vi "AutoWfmToSpreadsheet.vi"() -> ()   [LabVIEW 2017]
uses:
  <vilib>/Waveform/WDTOps.llb/WDT Scale Delta t DBL.vi
  <vilib>/Waveform/WDTFileIO.llb/Read Waveform from File.vi
  <vilib>/Waveform/WDTOps.llb/WDT Index Channel DBL.vi
  <vilib>/measure/maspectr.llb/FFT Power Spectrum and PSD for 1 Chan.vi
  <vilib>/Waveform/WDTFileIO.llb/Export Waveforms To Spreadsheet File (1D).vi
  <vilib>/measure/NI_MAPro.lvlib
panel:
  out "POWER":dbl[](graph)
  out "?":string
  out "Sinal adquirido":waveform(dbl)(graph)
  in  "?":bool
  in  "Escolher arquivo":i32
  out "Sinal de Referência":waveform(dbl)(graph)
  in  "Exportar":bool
  out "result string":string
  in  "Local da pasta com arquivos wfm":path=path "C:/Users/lucas/Documents/GitHub/INT/Novo Ensaio US/NOVOS_SINAIS/sinais/wfm"
  out "element":string
  out "Visualizar":i32
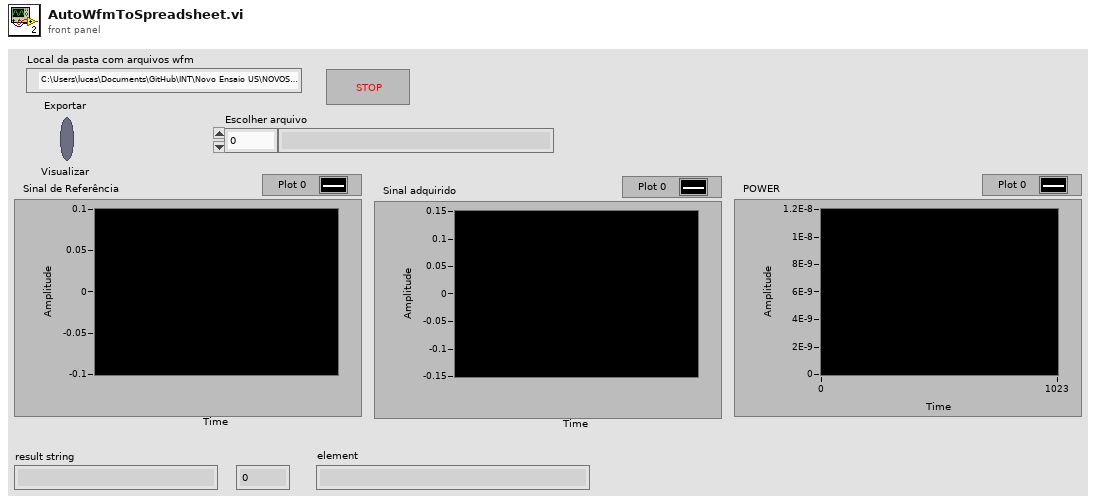
[diagram p1: front panel]
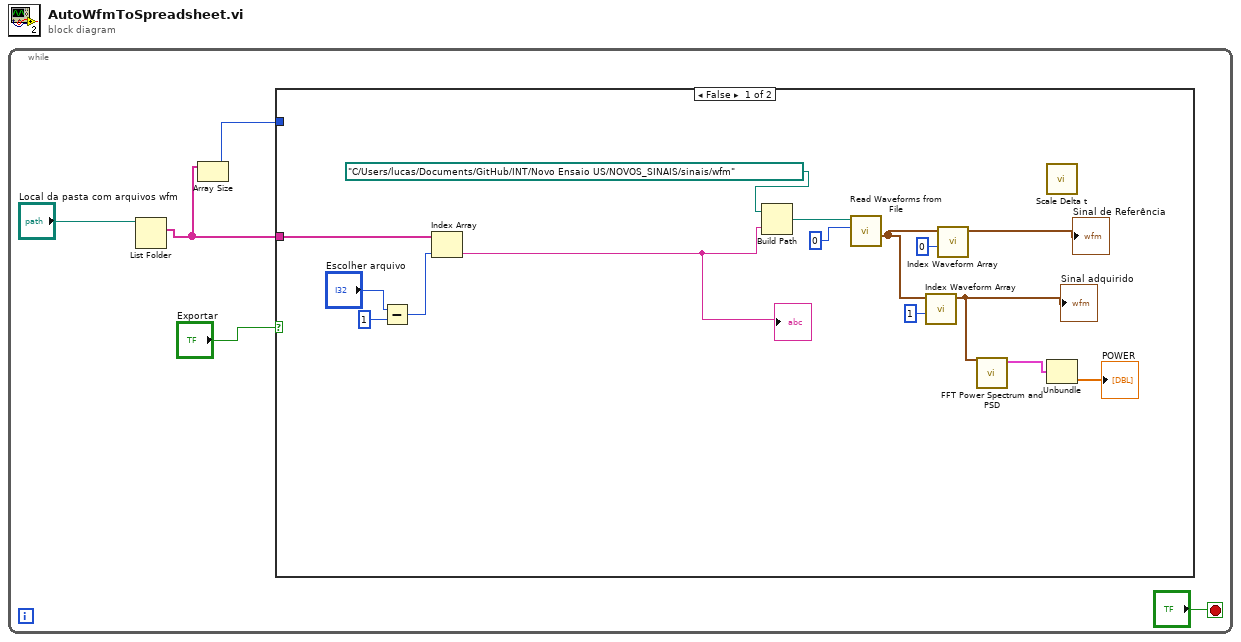
[diagram p0: block diagram]
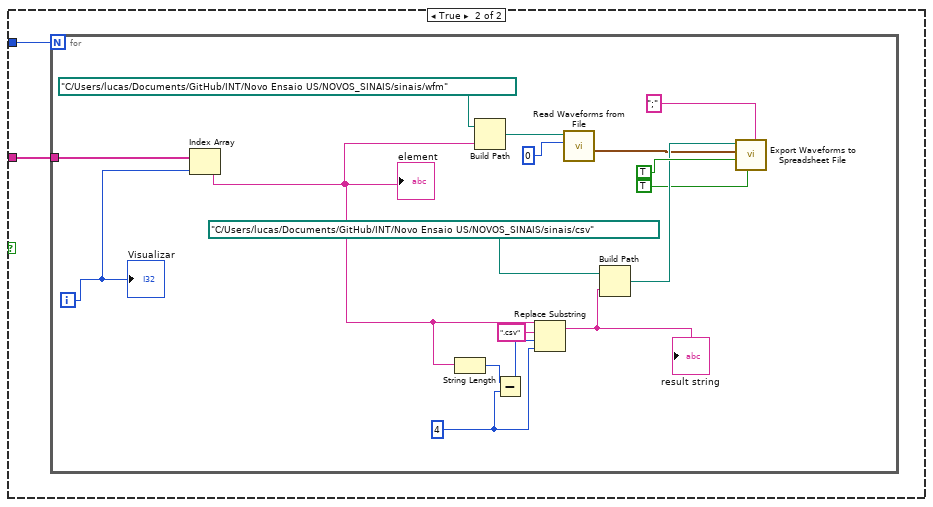
[diagram p2: hidden frame]
diagram:
  n1 = while {
    stop <- "?" stop-if-true
    n2 = List Folder(path="Local da pasta com arquivos wfm") -> (filenames=w4:string[])  [unwired: 3 in, 3 out]
    n3 = Array Size(array=w4) -> (size(s)=w3:i32)
    n4 = case shown="False" "Exportar" {
      tunnel: w4 -> [w17 w22]
      tunnel: w3 -> [_ w21]
      frame False {
        n5 = Subtract(x="Escolher arquivo", y=1) -> (x-y=w8:i32)
        n6 = Index Array(array=w17, index=w8) -> (element=w13:string)
        "?" <- w13
        n7 = Build Path(base path=path "C:/Users/lucas/Documents/GitHub/INT/Novo Ensaio US/NOVOS_SINAIS/sinais/wfm" ("file path (dialog if empty)"), name or relative path=w13) -> (appended path=w20:path)
        n8 = call-poly <vilib>:"Read Waveforms from File.vi"("offset (records:0)"=0, "file path (dialog if empty)"=w20) -> ("all waveforms in record"=w14:waveform(dbl)[])  [unwired: 4 in, 3 out]
        n9 = call-poly <vilib>:"Index Waveform Array.vi"("index"=1, "waveform array"=w14) -> ("waveform"=w9:waveform(dbl))  [unwired: 8 in, 1 out]
        "Sinal adquirido" <- w9
        n10 = call-poly <vilib>:"Index Waveform Array.vi"("index"=0, "waveform array"=w14) -> ("waveform"=→"Sinal de Referência":waveform(dbl))  [unwired: 8 in, 1 out]
        n11 = call-poly <vilib>:"FFT Power Spectrum and PSD.vi"("time signal"=w9) -> ("Power Spectrum / PSD"=w10:cluster{"f0":dbl, "df":dbl, "magnitude":dbl[]})  [unwired: 7 in, 3 out]
        n12 = call-poly <vilib>:"Scale Delta t.vi"() -> ()  [unwired: 10 in, 2 out]
        n13 = Unbundle(w10) -> ("magnitude"=→"POWER":dbl[])  [unwired: 2 out]
      }
      frame True {
        n14 = for {
          N: w21 -> [_]
          tunnel: w22 -> [w39]
          i -> [w38]
          w26 = 4 ("length (len. of substring)")
          n15 = Index Array(array=w39, index=w38) -> (element=w27:string)
          "element" <- w27
          n16 = String Length(string=w27) -> (length=w25:i32)
          n17 = Build Path(base path=path "C:/Users/lucas/Documents/GitHub/INT/Novo Ensaio US/NOVOS_SINAIS/sinais/wfm" ("file path (dialog if empty)"), name or relative path=w27) -> (appended path=w35:path)
          n18 = Subtract(x=w25, y=w26) -> (x-y=w24:i32)
          n19 = Replace Substring(2:w26, 3:w24, 4:".csv" ("substring (\"\")"), 5:w27) -> (1:w28:string)  [unwired: 1 out]
          "result string" <- w28
          n20 = call-poly <vilib>:"Read Waveforms from File.vi"("offset (records:0)"=0, "file path (dialog if empty)"=w35) -> ("all waveforms in record"=w23:waveform(dbl)[])  [unwired: 4 in, 3 out]
          n21 = Build Path(base path=path "C:/Users/lucas/Documents/GitHub/INT/Novo Ensaio US/NOVOS_SINAIS/sinais/csv" ("file path (dialog if empty)"), name or relative path=w28) -> (appended path=w31:path)
          n22 = call-poly <vilib>:"Export Waveforms to Spreadsheet File.vi"("delimiter (Tab)"=";", "append to file? (new file:F)"=TRUE, "multiple time columns? (single:F)"=TRUE, "waveforms"=w23, "file path (dialog if empty)"=w31) -> ()  [unwired: 5 in, 2 out]
          "Visualizar" <- w38
        }
      }
    }
  }
